vi "free_c_string_at_memory_address.vi"(8 "error in (no error)":errorcluster, 11 "memory_address":u64) -> (0 "error out":errorcluster)   [LabVIEW 2020]
uses:
  dragon_toml_64.dll
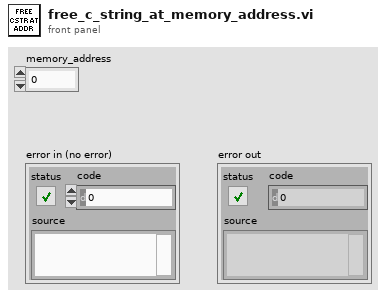
[diagram p1: front panel]
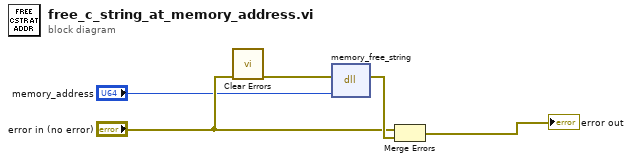
[diagram p0: block diagram]
diagram:
  n1 = call <vilib>:"Clear Errors.vi"("error in (no error)"="error in (no error)") -> ("error out"=w2:errorcluster)  [unwired: 5 in, 1 out]
  n2 = dll-call lib="C:/Projects/labview-project-load-tools/rust_src/toml_edit_dll/lv_src/dragon_toml_*.dll" fn="memory_free_string"(error in=w2, "ptr"="memory_address") -> (error out=w4:errorcluster)  [unwired: 4 in, 1 out]
  n3 = Merge Errors("error in (no error)", w4) -> (→"error out":errorcluster)
